vi "Connection to String.vi"(8 "error in":errorcluster, 9 "create module property if it doesn't exist? (T)":bool=TRUE, 10 "connection":T2, 11 "routing and faulting in":T1 format="%.0x") -> (0 "error out":errorcluster, 1 "conversion successful?":bool, 2 "string":string, 3 "routing and faulting out":T1 format="%.0x")   [LabVIEW 2020, in "Routing and Faulting Scripting.lvlib"]
uses:
  Routing and Faulting Scripting.lvlib
  Shared/Connection.ctl
  <vilib>/NI VeriStand/Custom Device API/Custom Device Item Ref.ctl
  Dependencies.llb/Routing and Faulting Shared.lvlib
  <vilib>/NI VeriStand/Custom Device API/Custom Device API.lvlib
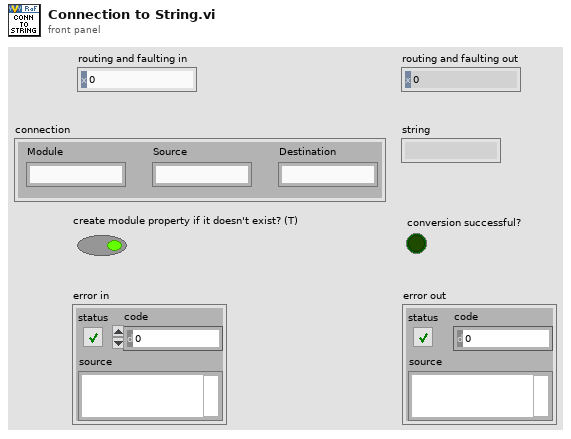
[diagram p1: front panel]
types:
  T1 = typedef "Custom Device API.lvlib/Custom Device Item Ref.ctl" = u64
  T2 = typedef "Routing and Faulting Shared.lvlib/Connection.ctl" = cluster{"Module":string, "Source":string, "Destination":string}
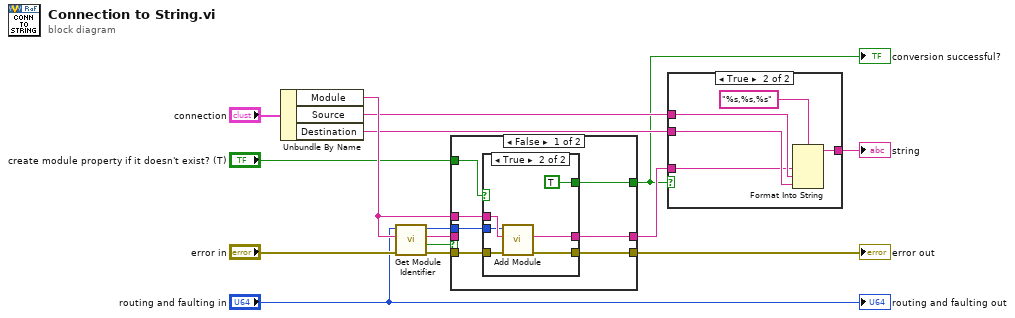
[diagram p0: block diagram]
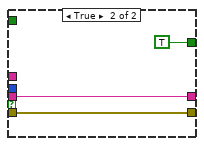
[diagram p4: hidden frame]
diagram:
  n1 = Unbundle By Name("connection") -> ("Module"=w10:string, "Source"=w8:string, "Destination"=w7:string)
  n2 = call "Get Module Identifier.vi"("error in"="error in", "module path"=w10, "routing and faulting in"="routing and faulting in") -> ("error out"=w13:errorcluster, "found?"=w14:bool, "module identifier"=w9:string, "routing and faulting out"=w11:T1)  [unwired: 5 in]
  n3 = case shown="False" w14 {
    tunnel: w13 -> [w22 w32]
    tunnel: [w19 w32] -> w12
    tunnel: w11 -> [w21 _]
    tunnel: w10 -> [w20 _]
    tunnel: w9 -> [_ w31]
    tunnel: [w18 w31] -> w5
    tunnel: "create module property if it doesn't exist? (T)" -> [w17 _]
    tunnel: [w16 TRUE] -> w3
    frame False {
      n4 = case shown="True" w17 {
        tunnel: w22 -> [w23 w24]
        tunnel: w21 -> [_ w25]
        tunnel: w20 -> [_ w29]
        tunnel: [w23 w28] -> w19
        tunnel: [_ w27] -> w18
        tunnel: [_ TRUE] -> w16
        frame False {
        }
        frame True {
          n5 = call "Add Module.vi"("error in"=w24, "module path"=w29, "routing and faulting in"=w25) -> ("error out"=w28:errorcluster, "unique module identifier"=w27:string)  [unwired: 6 in, 1 out]
        }
      }
    }
    frame True {
    }
  }
  "error out" <- w12
  "conversion successful?" <- w3
  n6 = case shown="True" w3 {
    tunnel: w8 -> [_ w37]
    tunnel: w7 -> [_ w36]
    tunnel: [_ w35] -> w6
    tunnel: w5 -> [_ w33]
    frame False {
    }
    frame True {
      n7 = Format Into String(format string="%s,%s,%s", w33, w37, w36) -> (resulting string=w35:string)  [unwired: 2 in, 1 out]
    }
  }
  "string" <- w6
  "routing and faulting out" <- "routing and faulting in"
